vi "GetPoint.vi"(8 "error in (no error)":errorcluster, 11 "Text in":refnum<class "Text.lvclass">) -> (0 "error out":errorcluster, 2 "Point":refnum<class "Point.lvclass">, 3 "Text out":refnum<class "Text.lvclass">)   [LabVIEW 2021]
uses:
  Text.lvclass
  Point1/Point.lvclass
  Text.lvclass/Text.ctl
  C:/Users/Dany/OneDrive/LabVIEW/Class/Picture2D/Shape/Shape.lvclass
  C:/Users/Dany/OneDrive/LabVIEW/Class/Picture2D/Picture2D/Picture2D.lvclass
  C:/Users/Dany/OneDrive/LabVIEW/Class/Picture2D/IDrawable/IDrawable.lvclass
  C:/Users/Dany/OneDrive/LabVIEW/Class/Picture2D/IMovable/IMovable.lvclass
  C:/Users/Dany/OneDrive/LabVIEW/Class/Picture2D/IRotatable/IRotatable.lvclass
  C:/Users/Dany/OneDrive/LabVIEW/Class/Picture2D/IScalable/IScalable.lvclass
  C:/Users/Dany/OneDrive/LabVIEW/Class/Picture2D/Text/Text.lvclass
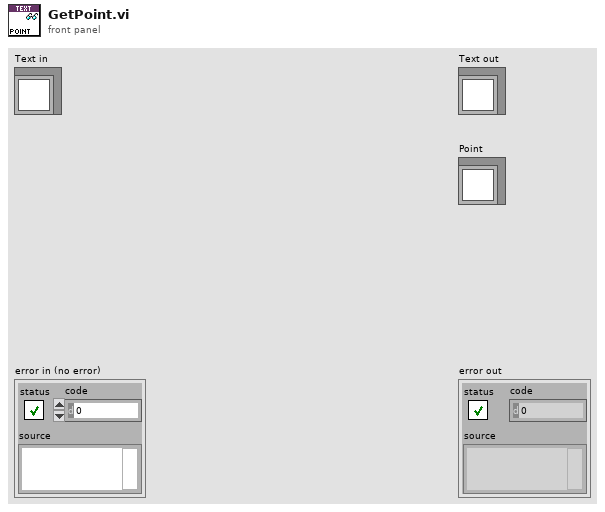
[diagram p1: front panel]
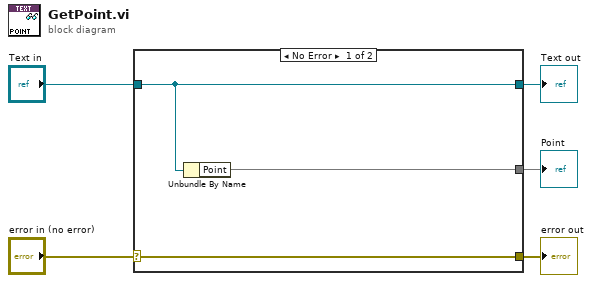
[diagram p0: block diagram]
diagram:
  n1 = case shown="No Error" "error in (no error)" {
    selector: "error in (no error)" -> [w8 w9]
    tunnel: [w8 w9] -> w4
    tunnel: [w7 w10] -> w2
    tunnel: "Text in" -> [w7 w10]
    tunnel: [w6 _] -> w1
    frame No Error {
      n2 = Unbundle By Name(w7) -> ("Point"=w6)
    }
    frame Error {
    }
  }
  "error out" <- w4
  "Text out" <- w2
  "Point" <- w1
